vi "DiffTest2.vi"() -> ()   [LabVIEW 2014]
panel:
  out "Boolean 2":bool
  in  "Boolean":bool
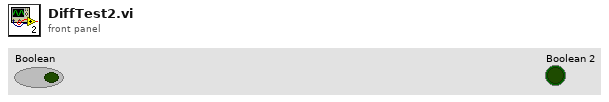
[diagram p1: front panel]
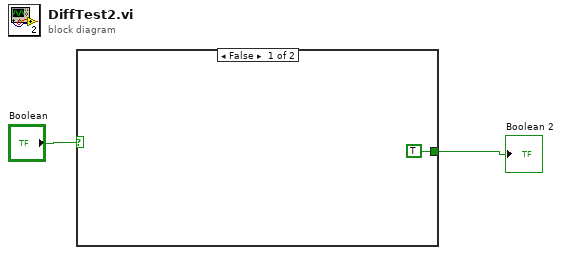
[diagram p0: block diagram]
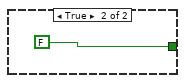
[diagram p2: hidden frame]
diagram:
  n1 = case shown="False" "Boolean" {
    tunnel: [TRUE FALSE] -> w1
    frame False {
    }
    frame True {
    }
  }
  "Boolean 2" <- w1
